vi "user32_SetMenu.vi"(0 "hWnd":u32, 5 "hMenu":u32, 11 "错误输入（无错误）":errorcluster) -> (4 "dup hWnd":u32, 6 "success?":bool, 15 "错误输出":errorcluster)   [LabVIEW 2011]
doc: "该函数分配一个新菜单到指定窗口。"
uses:
  user32.dll
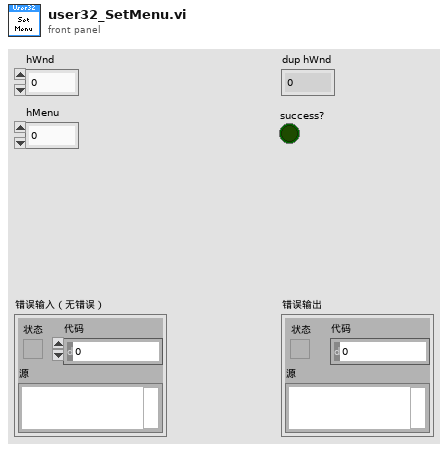
[diagram p1: front panel]
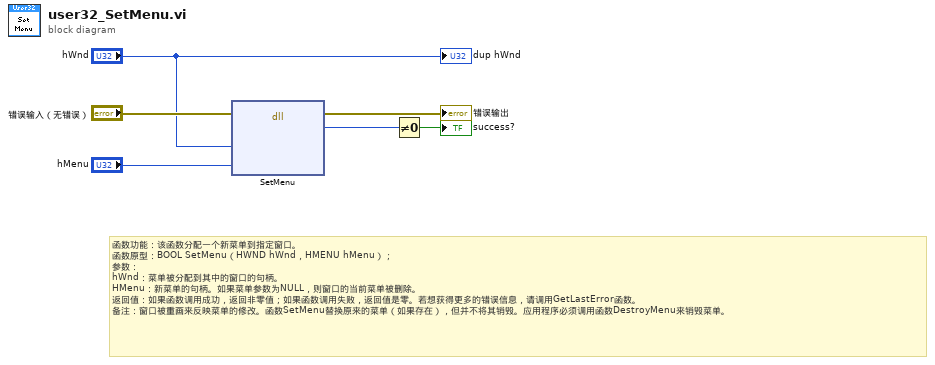
[diagram p0: block diagram]
diagram:
  # "函数功能：该函数分配一个新菜单到指定窗口。\n函数原型：BOOL SetMenu（HWND hWnd，HMENU hMenu）；\n参数：\nhWnd：菜单被分配到其中的窗口的句柄。\nHMenu：新菜单的句柄。如果菜单参数为NULL，则窗口的当前菜单被删除。\n返回值：如果函数调用成功，返回非零值；如果函数调用失败，返回值是零。若想获得更多的错误信息，请调用GetLastError函数。\n备注：窗口被重画来反映菜单的修改。函数SetMenu替换原来的菜单（如果存在），但并不将其销毁。应用程序必须调用函数DestroyMenu来销毁菜单。"
  n1 = dll-call lib="user32.dll" fn="SetMenu"(error in="错误输入（无错误）", "hWnd"="hWnd", "hMenu"="hMenu") -> (error out=→"错误输出":errorcluster, "Bool"=w3:u8)  [unwired: 4 in, 1 out]
  n2 = Not Equal To 0?(x=w3) -> (x != 0?=→"success?":bool)
  "dup hWnd" <- "hWnd"
